vi "RunAndExit.vi"   [LabVIEW 2013]
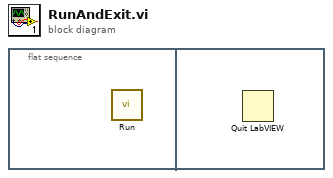
[diagram p0: block diagram]
diagram:
  n1 = flat-sequence {
    frame #0 {
      n2 = call "Run.vi"() -> ()  [unwired: 12 in]
    }
    frame #1 {
      n3 = Quit LabVIEW() -> ()  [unwired: 1 in]
    }
  }
